vi "edittest sequence form fields to records.vi"(8 "error in (no error)":errorcluster, 9 "fSpartanSetsSN":bool, 10 "Sequence FIELDs POST (empty)":T5, 11 "Connection Refnum":T1) -> (0 "error out":errorcluster, 2 "Sequence Fields":T2[](array[typedef]), 3 "Connection Refnum":T1)   [LabVIEW 2011]
uses:
  Addons/internet/utils/keyedarr.llb/Keyed Array.ctl
  server/database/Fields/Field Record.ctl
  server/database/Fields/Field DataTypes.ctl
  server/database/Fields/Field NextItem.ctl
  SI.LIB/ODBC/SQL Controls/Connection Refnum.ctl
panel:
  out "Debugging ... matches submitted fields with their respective attributes...":cluster{string, string}[](array[cluster])
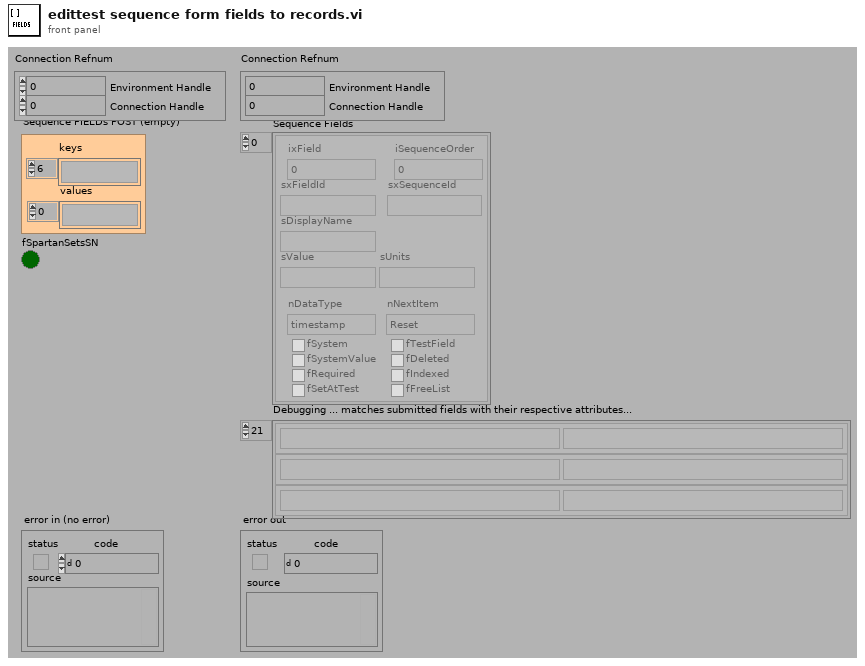
[diagram p1: front panel]
types:
  T1 = typedef "Connection Refnum.ctl" = cluster{"Environment Handle":i32, "Connection Handle":i32}
  T2 = typedef "Field Record.ctl" = cluster{"ixField":i32, "iSequenceOrder":i32, "sxFieldId":string, "sxSequenceId":string, "sDisplayName":string, "sValue":string, "sUnits":string, "nDataType":T3, "nNextItem":T4, "fSystem":bool, "fSystemValue":bool, "fRequired":bool, "fSetAtTest":bool, "fTestField":bool, "fDeleted":bool, "fIndexed":bool, "fFreeList":bool}
  T3 = typedef "Field DataTypes.ctl" = enum32{"text", "numeric", "list", "timestamp", "boolean"}
  T4 = typedef "Field NextItem.ctl" = enum32{"Reset", "Retain", "Auto-Increment"}
  T5 = typedef "Keyed Array.ctl" = cluster{"keys":string[], "values":string[]}
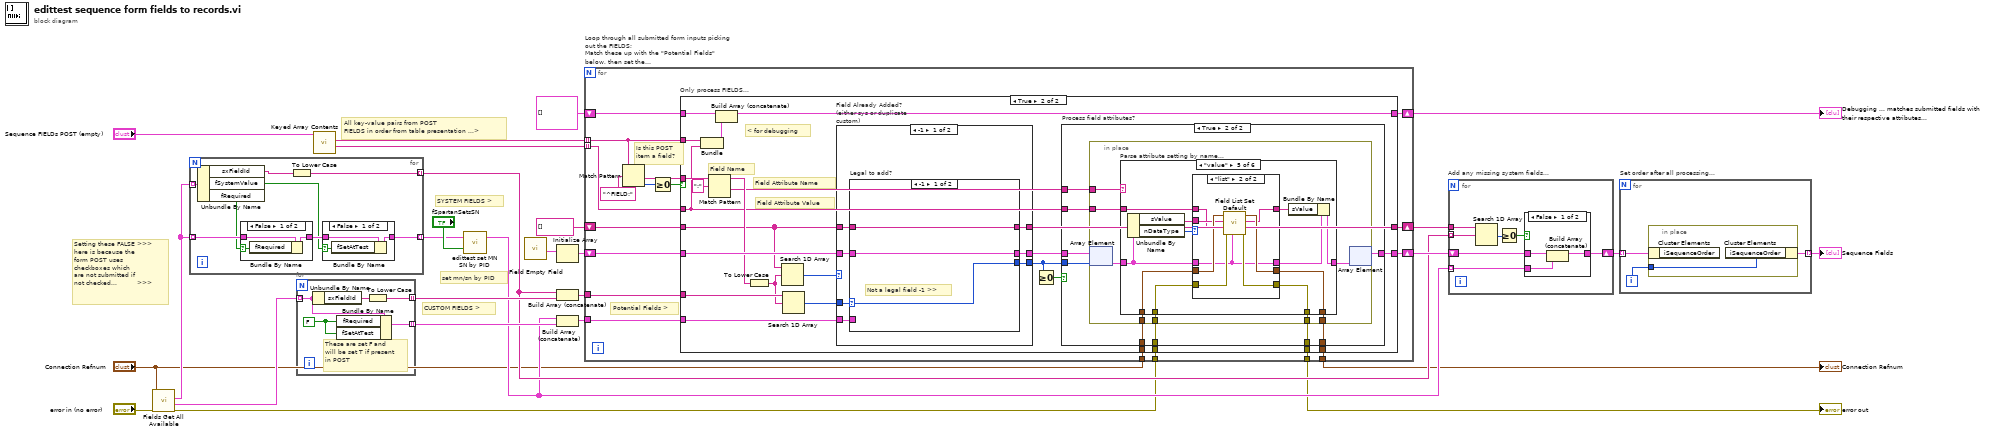
[diagram p0: block diagram]
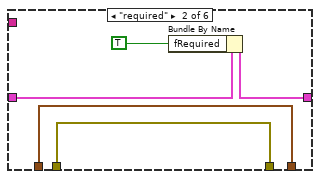
[diagram p8: hidden frame]
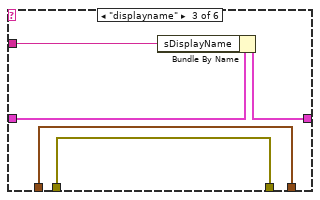
[diagram p9: hidden frame]
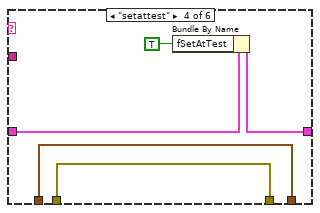
[diagram p10: hidden frame]
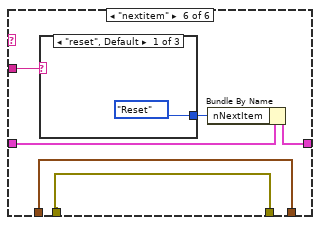
[diagram p12: hidden frame]
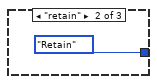
[diagram p13: hidden frame]
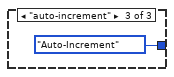
[diagram p14: hidden frame]
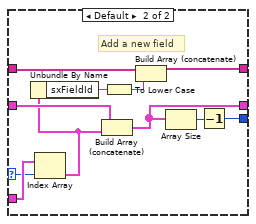
[diagram p15: hidden frame]
diagram:
  # "set mn/sn by PID"
  # "Setting these FALSE >>>\nhere is because the\nform POST uses\ncheckboxes which\nare not submitted if\nnot checked...          >>>"
  # "All key-value pairs from POST\nFIELDS in order from table presentation ...>"
  # "CUSTOM FIELDS >"
  # "SYSTEM FIELDS >"
  n1 = call "Fields Get All Available.vi"("error in (no error)"="error in (no error)", "Connection Refnum"="Connection Refnum") -> ("error out"=w4:errorcluster, "Custom Fields"=w5:T2[], "System or ALL Combined Fields"=w6:T2[])  [unwired: 3 in, 4 out]
  n2 = for {
    tunnel: w6 -> [w35] mode=indexing
    tunnel: [w33] -> w12 mode=indexing
    tunnel: w6 -> [w32] mode=indexing
    tunnel: [w29] -> w10 mode=indexing
    n3 = Unbundle By Name(w35) -> ("sxFieldId"=w34:string, "fSystemValue"=w28:bool, "fRequired"=w31:bool)
    n4 = case shown="False" w31 {
      selector: w31 -> [w40 _]
      tunnel: w32 -> [w42 w43]
      tunnel: [w41 w43] -> w30
      frame False {
        n5 = Bundle By Name(cluster=w42, "fRequired"=w40) -> (w41:T2)
      }
      frame True {
      }
    }
    n6 = To Lower Case(string=w34) -> (all lower case string=w33:string)
    n7 = case shown="False" w28 {
      selector: w28 -> [w36 _]
      tunnel: w30 -> [w38 w39]
      tunnel: [w37 w39] -> w29
      frame False {
        n8 = Bundle By Name(cluster=w38, "fSetAtTest"=w36) -> (w37:T2)
      }
      frame True {
      }
    }
  }
  n9 = for {
    tunnel: w5 -> [w46] mode=indexing
    tunnel: [w47] -> w17 mode=indexing
    tunnel: [w44] -> w16 mode=indexing
    w45 = FALSE
    # "These are set F and\nwill be set T if present\nin POST"
    n10 = Unbundle By Name(w46) -> ("sxFieldId"=w48:string)
    n11 = Bundle By Name(cluster=w46, "fRequired"=w45, "fSetAtTest"=w45) -> (w44:T2)
    n12 = To Lower Case(string=w48) -> (all lower case string=w47:string)
  }
  n13 = call "Keyed Array Contents.vi"("array in"="Sequence FIELDs POST (empty)") -> ("values"=w26:string[], "keys"=w27:string[])  [unwired: 5 out]
  n14 = call "edittest set MN SN by PID.vi"("fSpartanSetsSN"="fSpartanSetsSN", "FIELDS (empty)"=w10) -> ("FIELDS out"=w11:T2[])  [unwired: 1 out]
  n15 = call "Field Empty Field.vi"() -> ("Empty Field Record"=w21:T2)
  n16 = Initialize Array(w21) -> (w20:T2[])  [unwired: 1 out]
  n17 = Build Array (concatenate)(w12, w17) -> (w19:string[])
  n18 = Build Array (concatenate)(w11, w16) -> (w18:T2[])
  n19 = for "Loop through all submitted form inputs picking out the FIELDS;\nMatch these up with the \"Potential Fields\" below, then set the\nappropriate attributes as submitted in the form." {
    tunnel: w27 -> [w53] mode=indexing
    tunnel: w26 -> [w62] mode=indexing
    tunnel: w19 -> [w61]
    tunnel: w18 -> [w60]
    shift-right: [w57] -> w13
    shift-left: string[] [] -> [w59]
    shift-right: [w56] -> w15
    shift-left: w20 -> [w58]
    shift-right: [w54] -> w9
    shift-left: cluster{string, string}[] [] ("Array") -> [w55]
    tunnel: w4 -> [w52]
    tunnel: [w51] -> w3
    tunnel: "Connection Refnum" -> [w50]
    tunnel: [w49] -> w1
    # "Potential Fields >"
    # "Is this POST\nitem a field?"
    n20 = Match Pattern(string=w53, regular expression="^FIELD:") -> (after substring=w64:string, offset past match=w65:i32)  [unwired: 3 out]
    n21 = Greater Or Equal To 0?(x=w65) -> (x >= 0?=w63:bool)
    n22 = case "Only process FIELDS..." shown="True" w63 {
      tunnel: w64 -> [_ w81]
      tunnel: w58 -> [w71 w96]
      tunnel: [w71 w85] -> w56
      tunnel: w62 -> [_ w77]
      tunnel: w59 -> [w70 w93]
      tunnel: [w70 w88] -> w57
      tunnel: w61 -> [_ w92]
      tunnel: w60 -> [_ w89]
      tunnel: w55 -> [w69 w82]
      tunnel: [w69 w80] -> w54
      tunnel: w53 -> [_ w79]
      tunnel: w52 -> [w68 w75]
      tunnel: [w68 w74] -> w51
      tunnel: w50 -> [w67 w73]
      tunnel: [w67 w72] -> w49
      frame False {
        # "POST item is not a field - skip processing..."
      }
      frame True {
        # "< for debugging"
        # "Field Attribute Value"
        # "Field Attribute Name"
        # "Field Name"
        n23 = Bundle(w79, w77) -> (w78:cluster{string, string})  [unwired: 1 out]
        n24 = Match Pattern(string=w81, regular expression=":") -> (before substring=w94:string, after substring=w83:string)  [unwired: 3 out]
        n25 = Build Array (concatenate)(w82, w78) -> (w80:cluster{string, string}[])
        n26 = To Lower Case(string=w94) -> (all lower case string=w91:string)
        n27 = Search 1D Array(1D array=w93, element=w91) -> (index of element=w76:i32)  [unwired: 1 out]
        n28 = Search 1D Array(1D array=w92, element=w91) -> (index of element=w90:i32)  [unwired: 1 out]
        n29 = case "Field Already Added? (either sys or duplicate custom)" shown="-1" w76 {
          selector: w76 -> [_ w188]
          tunnel: w96 -> [w173 w189]
          tunnel: [w172 w189] -> w87
          tunnel: w93 -> [w171 w190]
          tunnel: [w170 w190] -> w88
          tunnel: w90 -> [w167 _]
          tunnel: w89 -> [w169 _]
          tunnel: [w168 w188] -> w84
          frame -1 {
            n30 = case "Legal to add?" shown="-1" w167 {
              selector: w167 -> [w174 w177]
              tunnel: w173 -> [w176 w182]
              tunnel: [w176 w180] -> w172
              tunnel: w171 -> [w175 w185]
              tunnel: [w175 w184] -> w170
              tunnel: w169 -> [_ w187]
              tunnel: [w174 w178] -> w168
              frame -1 {
                # "Not a legal field -1 >>"
              }
              frame Default {
                # "Add a new field"
                n31 = Index Array(array=w187, index=w177) -> (element=w181:T2)
                n32 = Unbundle By Name(w181) -> ("sxFieldId"=w186:string)
                n33 = Build Array (concatenate)(w182, w181) -> (w180:T2[])
                n34 = To Lower Case(string=w186) -> (all lower case string=w183:string)
                n35 = Build Array (concatenate)(w185, w183) -> (w184:string[])
                n36 = Array Size(array=w180) -> (size(s)=w179:i32)
                n37 = Decrement(x=w179) -> (x-1=w178:i32)
              }
            }
          }
          frame Default {
          }
        }
        n38 = Greater Or Equal To 0?(x=w84) -> (x >= 0?=w86:bool)
        n39 = case "Process field attributes?" shown="True" w86 {
          tunnel: w87 -> [w99 w108]
          tunnel: [w99 w107] -> w85
          tunnel: w84 -> [_ w104]
          tunnel: w83 -> [_ w106]
          tunnel: w77 -> [_ w105]
          tunnel: w75 -> [w98 w103]
          tunnel: [w98 w102] -> w74
          tunnel: w73 -> [w97 w101]
          tunnel: [w97 w100] -> w72
          frame False {
          }
          frame True {
            n40 = in-place {
              in-place-border: w106 -> [w115]
              in-place-border: w105 -> [w113]
              in-place-border: w103 -> [w112]
              in-place-border: [w111] -> w102
              in-place-border: w101 -> [w110]
              in-place-border: [w109] -> w100
              n41 = in-place-array #1(w108, w104) -> (w116:T2)
              n42 = case "Parse attribute setting by name..." shown="\"value\"" w115 {
                tunnel: w116 -> [w119 w123 w128 w134 w136 w163]
                tunnel: [w119 w124 w129 w133 w145 w162] -> w114
                tunnel: w113 -> [_ _ w127 _ w143 w161]
                tunnel: w112 -> [w118 w121 w126 w131 w140 w159]
                tunnel: [w118 w121 w126 w131 w139 w159] -> w111
                tunnel: w110 -> [w117 w120 w125 w130 w138 w158]
                tunnel: [w117 w120 w125 w130 w137 w158] -> w109
                frame "UNKNOWN", Default {
                }
                frame "required" {
                  n43 = Bundle By Name(cluster=w123, "fRequired"=TRUE) -> (w124:T2)
                }
                frame "displayname" {
                  n44 = Bundle By Name(cluster=w128, "sDisplayName"=w127) -> (w129:T2)
                }
                frame "setattest" {
                  n45 = Bundle By Name(cluster=w134, "fSetAtTest"=TRUE) -> (w133:T2)
                }
                frame "value" {
                  n46 = Unbundle By Name(w136) -> ("sValue"=w141:string, "nDataType"=w142:T3)
                  n47 = case shown="\"list\"" w142 {
                    tunnel: [w149 w153] -> w144
                    tunnel: w143 -> [w149 w151]
                    tunnel: w141 -> [_ w152]
                    tunnel: w140 -> [w148 w157]
                    tunnel: [w148 w156] -> w139
                    tunnel: w138 -> [w147 w155]
                    tunnel: [w147 w154] -> w137
                    tunnel: w136 -> [w146 w150]
                    tunnel: [w146 w150] -> w135
                    frame "text", Default {
                    }
                    frame "list" {
                      n48 = call "Field List Set Default.vi"("FIELD (empty)"=w150, "error in (no error)"=w157, "Default Value (\"\")"=w151, "Flat List (\"\")"=w152, "Connection Refnum"=w155) -> ("error out"=w156:errorcluster, "New Flat List"=w153:string, "dup Connection Refnum"=w154:T1)  [unwired: 4 out]
                    }
                  }
                  n49 = Bundle By Name(cluster=w135, "sValue"=w144) -> (w145:T2)
                }
                frame "nextitem" {
                  n50 = case shown="\"reset\", Default" w161 {
                    tunnel: [Field_NextItem."Reset" ("nNextItem") Field_NextItem."Retain" ("nNextItem") Field_NextItem."Auto-Increment" ("nNextItem")] -> w160
                    frame "reset", Default {
                    }
                    frame "retain" {
                    }
                    frame "auto-increment" {
                    }
                  }
                  n51 = Bundle By Name(cluster=w163, "nNextItem"=w160) -> (w162:T2)
                }
              }
              n52 = in-place-array #1(w114) -> (w107:T2[])  [unwired: 1 out]
            }
          }
        }
      }
    }
  }
  "error out" <- w3
  "Connection Refnum" <- w1
  "Debugging ... matches submitted fields with their respective attributes..." <- w9
  n53 = for "Add any missing system fields..." {
    shift-right: [w191] -> w14
    shift-left: w15 -> [w194]
    tunnel: w13 -> [w197]
    tunnel: w12 -> [w196] mode=indexing
    tunnel: w11 -> [w195] mode=indexing
    n54 = Search 1D Array(1D array=w197, element=w196) -> (index of element=w193:i32)  [unwired: 1 out]
    n55 = Greater Or Equal To 0?(x=w193) -> (x >= 0?=w192:bool)
    n56 = case shown="False" w192 {
      tunnel: w195 -> [w198 _]
      tunnel: w194 -> [w200 w201]
      tunnel: [w199 w201] -> w191
      frame False {
        n57 = Build Array (concatenate)(w200, w198) -> (w199:T2[])
      }
      frame True {
      }
    }
  }
  n58 = for "Set order after all processing..." {
    tunnel: w14 -> [w204] mode=indexing
    tunnel: [w202] -> w24 mode=indexing
    i -> [w203]
    n59 = in-place {
      in-place-border: w203 -> [w205]
      n60 = in-place-cluster #2(w204) -> ()  [unwired: 1 out]
      n61 = in-place-cluster #2("iSequenceOrder"=w205) -> (w202:T2)
    }
  }
  "Sequence Fields" <- w24
